vi "Execute Displayed Sequence.vi"(5 "Break at First Step? (F)":bool, 6 "Process Model (Default)":refnum<class "SequenceFile.lvclass">, 7 "Execution Options (Default)":T1={"Use Default Model (T)"=TRUE, "Release Related References (T)"=TRUE}, 8 "error in (no error)":errorcluster, 10 "Entry Point":string="Single Pass", 11 "SequenceViewPanel in":refnum<class "SequenceViewPanel.lvclass">) -> (0 "error out":errorcluster, 2 "Execution":refnum<class "Execution.lvclass">, 3 "SequenceViewPanel out":refnum<class "SequenceViewPanel.lvclass">)   [LabVIEW 2020, in "TSnax UI.lvlib" / "SequenceViewPanel.lvclass"]
uses:
  SequenceViewPanel.lvclass
  SequenceViewPanel.lvclass/SequenceViewPanel.ctl
  TSnax/Execution/Execution.lvclass
  TSnax/Execution Options.ctl
  TSnax/TSnax.lvlib
  TSnax/SequenceFile/SequenceFile.lvclass
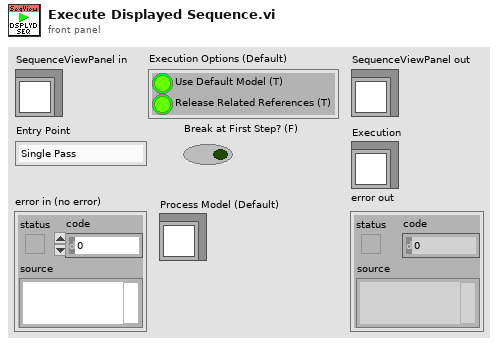
[diagram p1: front panel]
types:
  T1 = typedef "TSnax.lvlib/Execution Options.ctl" = cluster{"Use Default Model (T)":bool, "Release Related References (T)":bool}
  T2 = typedef "TSnax UI.lvlib/SequenceViewPanel.lvclass/Ref Data.ctl" = cluster{"Insert Line":i32, "SequenceFile":refnum<class "SequenceFile.lvclass">, "Sequence":string, "Trace Marker":i32, "Execution":refnum<class "Execution.lvclass">}
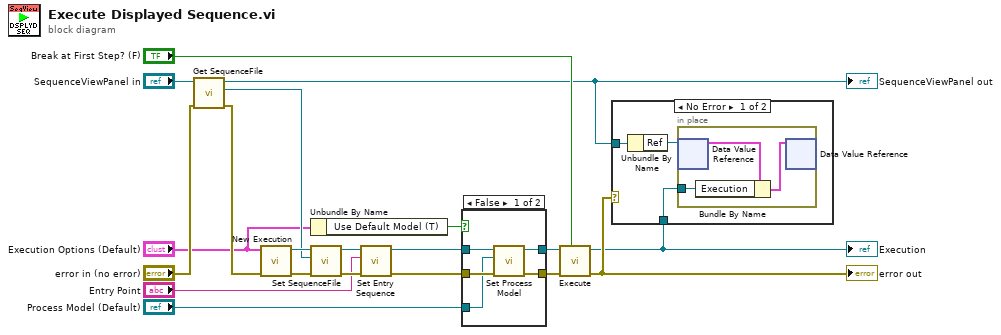
[diagram p0: block diagram]
diagram:
  n1 = call "Get SequenceFile.vi"("error in (no error)"="error in (no error)", "SequenceViewPanel in"="SequenceViewPanel in") -> ("error out"=w11:errorcluster, "SequenceFile"=w13:refnum<class "SequenceFile.lvclass">, "SequenceViewPanel out"=w2:refnum<class "SequenceViewPanel.lvclass">)  [unwired: 7 in]
  "SequenceViewPanel out" <- w2
  n2 = call "New Execution.vi"("error in (no error)"=w11, "Execution Options (Default)"="Execution Options (Default)") -> ("error out"=w18:errorcluster, "Execution out"=w19:refnum<class "Execution.lvclass">)  [unwired: 8 in]
  n3 = Unbundle By Name("Execution Options (Default)") -> ("Use Default Model (T)"=w6:bool)
  n4 = call "Set SequenceFile.vi"("error in (no error)"=w18, "SequenceFile"=w13, "Execution in"=w19) -> ("error out"=w16:errorcluster, "Execution out"=w17:refnum<class "Execution.lvclass">)  [unwired: 7 in]
  n5 = call "Set Entry Sequence.vi"("error in (no error)"=w16, "Entry Sequence"="Entry Point", "Execution in"=w17) -> ("error out"=w10:errorcluster, "Execution out"=w9:refnum<class "Execution.lvclass">)  [unwired: 7 in]
  n6 = case shown="False" w6 {
    tunnel: w10 -> [w24 w26]
    tunnel: w9 -> [w25 w27]
    tunnel: "Process Model (Default)" -> [w23 _]
    tunnel: [w21 w27] -> w5
    tunnel: [w22 w26] -> w4
    frame False {
      n7 = call "Set Process Model.vi"("error in (no error)"=w24, "Process Model"=w23, "Execution in"=w25) -> ("error out"=w22:errorcluster, "Execution out"=w21:refnum<class "Execution.lvclass">)  [unwired: 7 in]
    }
    frame True {
    }
  }
  n8 = call "Execute.vi"("Break at First Step? (F)"="Break at First Step? (F)", "error in (no error)"=w4, "Execution in"=w5) -> ("error out"=w20:errorcluster, "Execution out"=w1:refnum<class "Execution.lvclass">)  [unwired: 7 in]
  "error out" <- w20
  "Execution" <- w1
  n9 = case shown="No Error" w20 {
    tunnel: w2 -> [w29 _]
    tunnel: w1 -> [w28 _]
    frame No Error {
      n10 = Unbundle By Name(w29) -> ("Ref"=w30:refnum<data-value>)
      n11 = in-place {
        in-place-border: w28 -> [w31]
        n12 = in-place-dvr #1(w30) -> (w33:T2)  [unwired: 1 out]
        n13 = Bundle By Name(cluster=w33, "Execution"=w31) -> (w32:T2)
        n14 = in-place-dvr #1(w32) -> ()  [unwired: 2 out]
      }
    }
    frame Error {
    }
  }
